vi "Create Cancellation Token.vi"(7 "IncludeTimeout (T)":bool=TRUE, 8 "error in (no error)":errorcluster, 11 "Timeout_ms (10000)":i32=10000) -> (0 "error out":errorcluster, 2 "NET_CancellationSource":refnum<k24>, 3 "NET_CancellationToken":refnum<k24>)   [LabVIEW 2018, in "LabVIEWHTTPClient_NET.lvlib" / "LabVIEWHTTPClient_NET.lvclass"]
uses:
  LabVIEWHTTPClient_NET.lvclass
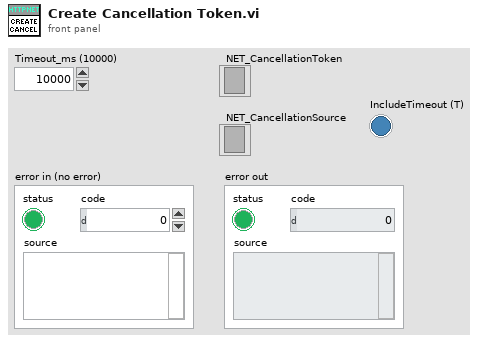
[diagram p1: front panel]
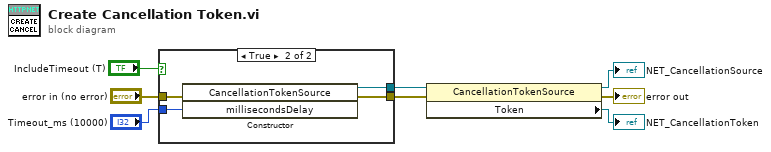
[diagram p0: block diagram]
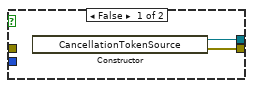
[diagram p2: hidden frame]
diagram:
  n1 = case shown="True" "IncludeTimeout (T)" {
    tunnel: "Timeout_ms (10000)" -> [_ w11]
    tunnel: [w10 w14] -> w4
    tunnel: "error in (no error)" -> [_ w13]
    tunnel: [w9 w12] -> w1
    frame False {
      n2 = constructor class="CancellationTokenSource"() -> (reference out=w9:refnum<k24>, error out=w10:errorcluster)  [unwired: 3 in, 1 out]
    }
    frame True {
      n3 = constructor class="CancellationTokenSource"(error in=w13, "millisecondsDelay"=w11) -> (reference out=w12:refnum<k24>, error out=w14:errorcluster)  [unwired: 2 in, 2 out]
    }
  }
  n4 = property class="CancellationTokenSource"(reference=w1, error in=w4) -> (reference out=→"NET_CancellationSource":refnum<k24>, error out=→"error out":errorcluster, "Token"=→"NET_CancellationToken":refnum<k24>)
